vi "Transform.vi"(7 "Type X":T1(ring), 8 "error in (no error)":errorcluster caption="entrée d'erreur (pas d'erreur)", 9 "y":string[][](array[string]), 10 "X":string[][](array[string]), 11 "RobustScaler.lvclass":refnum<class "RobustScaler.lvclass">) -> (0 "error out":errorcluster caption="sortie d'erreur", 2 "Data":T2, 3 "RobustScaler.lvclass":refnum<class "RobustScaler.lvclass">)   [LabVIEW 2020, in "RobustScaler.lvclass"]
doc: "Center and scale the data.\n\nReturns : \n\n- X_new : ndarray array of shape (n_samples, n_features_new)\nTransformed array."
uses:
  RobustScaler.lvclass
  RobustScaler.lvclass/RobustScaler.ctl
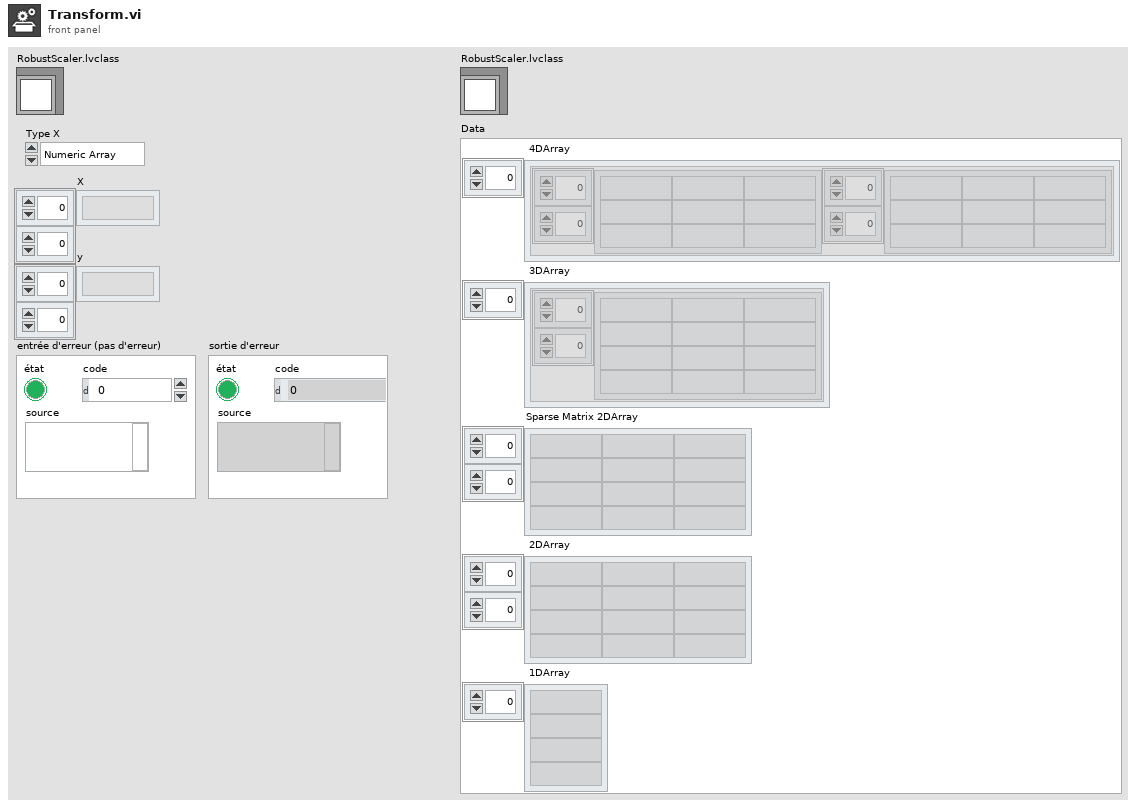
[diagram p1: front panel]
types:
  T1 = enum16{"Numeric Array", "String Array", "Sparse"}
  T2 = cluster{" 4DArray":cluster{"1":string[][], "2":string[][]}[], " 3DArray":cluster{"Tableau":string[][]}[], "Sparse Matrix 2DArray":string[][], " 2DArray":string[][], " 1DArray":string[]}
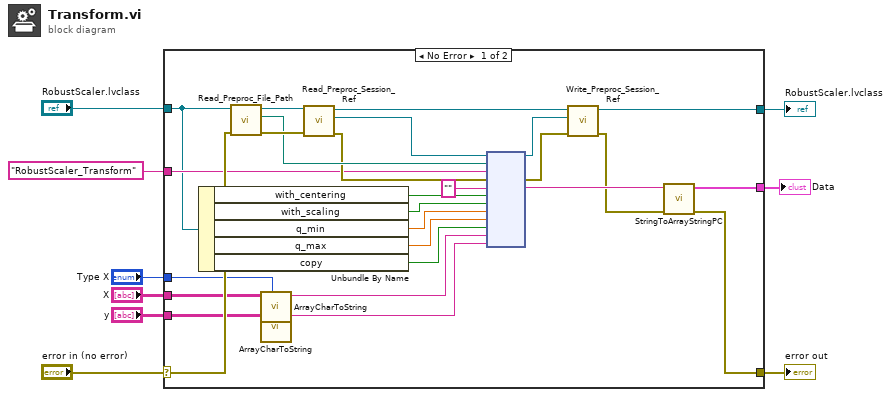
[diagram p0: block diagram]
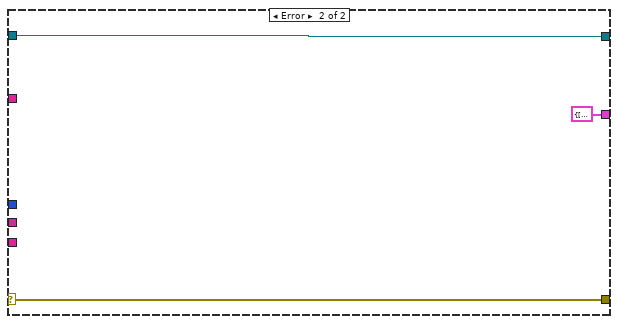
[diagram p2: hidden frame]
diagram:
  n1 = case shown="No Error" "error in (no error)" {
    selector: "error in (no error)" -> [w24 w39]
    tunnel: [w16 w39] -> w8
    tunnel: [w18 w38] -> w6
    tunnel: "RobustScaler.lvclass" -> [w22 w38]
    tunnel: "RobustScaler_Transform" ("Fonction") -> [w23 _]
    tunnel: [w15 T2 {" 4DArray"=[], " 3DArray"=[], "Sparse Matrix 2DArray"=[], " 2DArray"=[], " 1DArray"=[]} ("Data")] -> w4
    tunnel: "X" -> [w14 _]
    tunnel: "y" -> [w13 _]
    tunnel: "Type X" -> [w12 _]
    frame No Error {
      n2 = Unbundle By Name(w22) -> ("with_centering"=w27:bool, "with_scaling"=w26:bool, "q_min"=w25:dbl, "q_max"=w21:dbl, "copy"=w20:bool)
      n3 = call-dynamic "Read_Preproc_File_Path.vi"("error in (no error)"=w24, "Python in"=w22) -> ("error out"=w35:errorcluster, "File_Path"=w32:path, "Python out"=w36:refnum<class "RobustScaler.lvclass">)  [unwired: 7 in]
      n4 = call "ArrayCharToString.vi"("Type"=w12, "TAB"=w14) -> ("Instruction"=w11:string)  [unwired: 9 in]
      n5 = call "ArrayCharToString.vi"("TAB"=w13) -> ("Instruction"=w10:string)  [unwired: 10 in]
      n6 = call-dynamic "Read_Preproc_Session_Ref.vi"("error in (no error)"=w35, "Python in"=w36) -> ("error out"=w31:errorcluster, "Session_ref"=w33:refnum<k35>, "Python out"=w34:refnum<class "RobustScaler.lvclass">)  [unwired: 7 in]
      n7 = node(w33, w32, w23, w31, "", w27, w26, w25, w21, w20, w11, w10) -> (w29:refnum<k35>, w30:errorcluster, w19:string)  [unwired: 7 in, 2 out]
      n8 = call-dynamic "Write_Preproc_Session_Ref.vi"("error in (no error)"=w30, "Session_ref"=w29, "Python in"=w34) -> ("error out"=w17:errorcluster, "Python out"=w18:refnum<class "RobustScaler.lvclass">)  [unwired: 7 in]
      n9 = call "StringToArrayStringPC.vi"("sortie d'erreur"=w17, "Return value"=w19) -> ("sortie d'erreur"=w16:errorcluster, "Data"=w15:T2)  [unwired: 8 in]
    }
    frame Error {
    }
  }
  "error out" <- w8
  "RobustScaler.lvclass" <- w6
  "Data" <- w4
